vi "My Nonlinear Curve Fit TRDL bounds.vi"(0 "Y":dbl[](array[numeric]), 1 "f(x,a)":T5, 2 "data":variant, 5 "X":dbl[](array[numeric]), 7 "Weight":dbl[](array[numeric]), 9 "initial parameters":dbl[](array[numeric]), 11 "error in (no error)":errorcluster, 12 "Termination Criteria":T6={"Max Iterations"=0, "Max Function Calls"=0, "Max Time"=1000.0, "Function Tolerance"=1e-06, "Parameter Tolerance"=1e-06, "Gradient Tolerance"=0.0, "Min Lambda"=1e-06, "Max Lambda"=1e-06, "Initial Tick Count"=0}, 13 "parameter bounds":T4, 14 "method":T3 items=["Least Square", "Least Absolute Residual", "Bisquare"]) -> (3 "Fit Aborted?":bool, 4 "best nonlinear fit":dbl[](array[numeric]), 6 "best fit parameters":dbl[](array[numeric]), 8 "covariance":T7, 10 "Fit Statistics":T1={"# Iterations"=0, "# Function Calls"=0, "Chi2"=0.0, "Chi2/DOF"=0.0, "Fit Convergence Criterion"=enum."Continue", "Gradient"=0.0, "|Delta Chi 2|"=0.0, "|Delta Chi 2|/Chi 2"=0.0, "Max |Delta a| /|a|"=0.0, "Lambda"=-1.0}, 15 "error out":errorcluster)   [LabVIEW 2021, in "Fits.lvlib"]
uses:
  Fits.lvlib
  <vilib>/gmath/NumericalOptimization/LM_output select.ctl
  <vilib>/gmath/NI_Gmath.lvlib
  <vilib>/Analysis/NI_AALBase.lvlib
  <vilib>/gmath/NumericalOptimization/LM model function reference.ctl
  <vilib>/gmath/NumericalOptimization/LM model function.ctl
  Fit Statistics v3.ctl
  Abort Fit Global.vi
  <vilib>/Analysis/baseanly.llb/Real Inverse Matrix.vi
  Error/Error.lvlib
  Convergence Criteria.ctl
  <vilib>/Analysis/Matrix/Datatypes/RealMatrix.ctl
  <vilib>/Analysis/Matrix/NI_Matrix.lvlib
  <vilib>/Analysis/6fits.llb/Curve Fitting Criteria.ctl
  <vilib>/Analysis/NI_AALPro.lvlib
  My Fit Stopping Criteria.ctl
panel:
  out "Waveform Graph":dbl[](graph)
  in  "Delay (ms)":i32
  in  "Debug":bool
  out "Parameters Chart":dbl[][](graph)
  out "Function & Fit Graph":cluster{"New Coefficients":dbl[]}[](graph)
  in  "TR update constants":cluster{"h1":dbl, "h2":dbl, "a1":dbl, "a2":dbl}={"h1"=0.0001, "h2"=0.99, "a1"=0.25, "a2"=3.5}
  out "number of function calls":i32
  out "residue":dbl
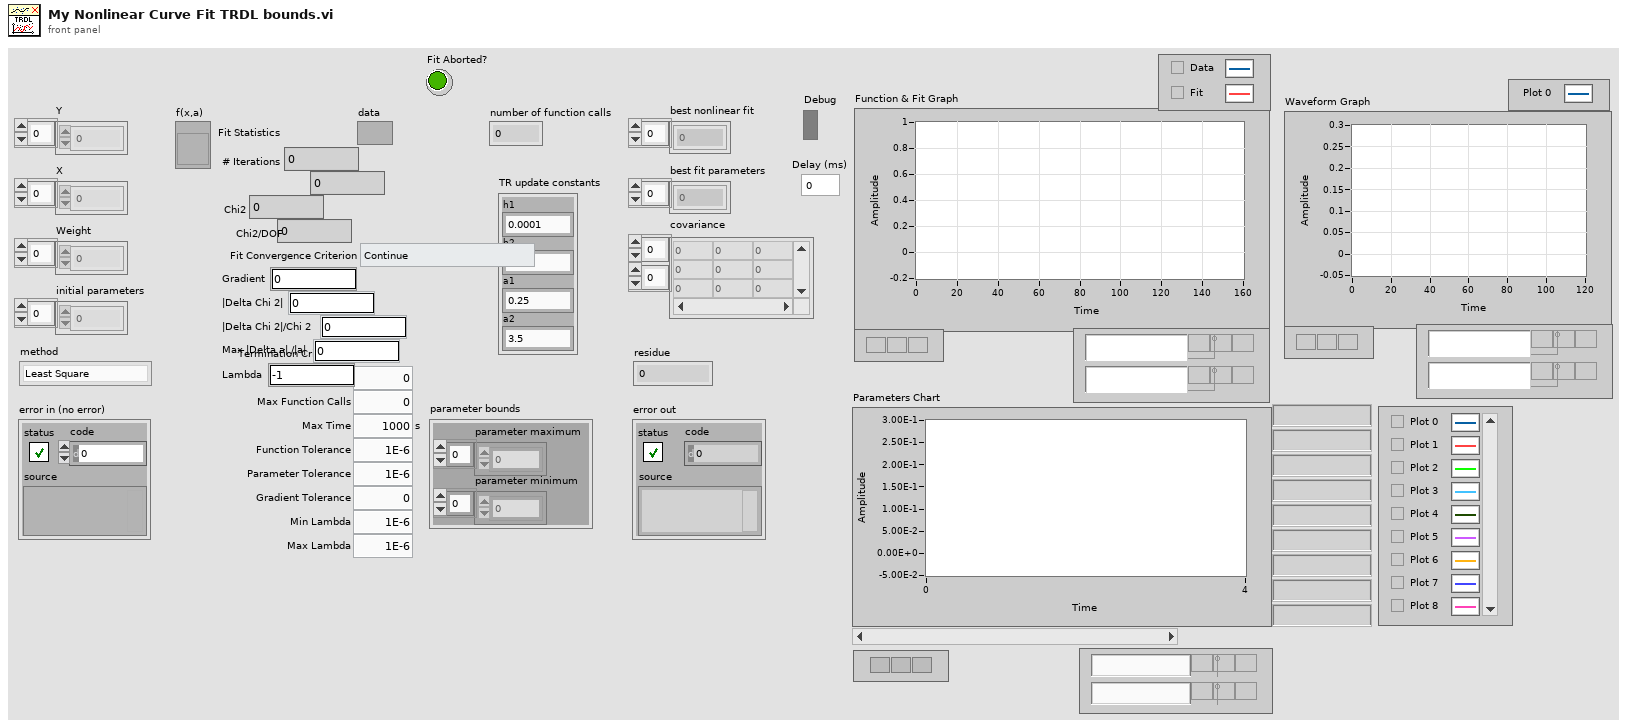
[diagram p1: front panel]
types:
  T1 = typedef "Fits.lvlib/Fit Statistics v2.ctl" = cluster{"# Iterations":i32, "# Function Calls":i32, "Chi2":dbl, "Chi2/DOF":dbl, "Fit Convergence Criterion":T2, "Gradient":dbl, "|Delta Chi 2|":dbl, "|Delta Chi 2|/Chi 2":dbl, "Max |Delta a| /|a|":dbl, "Lambda":dbl}
  T2 = typedef "Fits.lvlib/Convergence Criteria.ctl" = enum16{"Continue", "Tolerances Exceeded", "Max Time Exceeded", "Max Iterations Exceeded", "Max Function Evaluations Exceeded", "Scale Range Exceeded"}
  T3 = typedef "NI_AALPro.lvlib/Curve Fitting Criteria.ctl" = u16
  T4 = cluster{"parameter minimum":dbl[], "parameter maximum":dbl[]}
  T5 = typedef "NI_Gmath.lvlib/LM model function reference.ctl" = refnum<vi>
  T6 = typedef "Fits.lvlib/My Fit Stopping Criteria.ctl" = cluster{"Max Iterations":i32, "Max Function Calls":i32, "Max Time":dbl[unit], "Function Tolerance":dbl, "Parameter Tolerance":dbl, "Gradient Tolerance":dbl, "Min Lambda":dbl, "Max Lambda":dbl, "Initial Tick Count":u32}
  T7 = typedef "NI_Matrix.lvlib/RealMatrix.ctl" = dbl[][]
  T8 = typedef "NI_Gmath.lvlib/LM model function.ctl" = cluster{"f(x,a)":T5, "data":variant}
  T9 = typedef "NI_Gmath.lvlib/LM_output select.ctl" = cluster{"model function":bool, "gradient":bool}
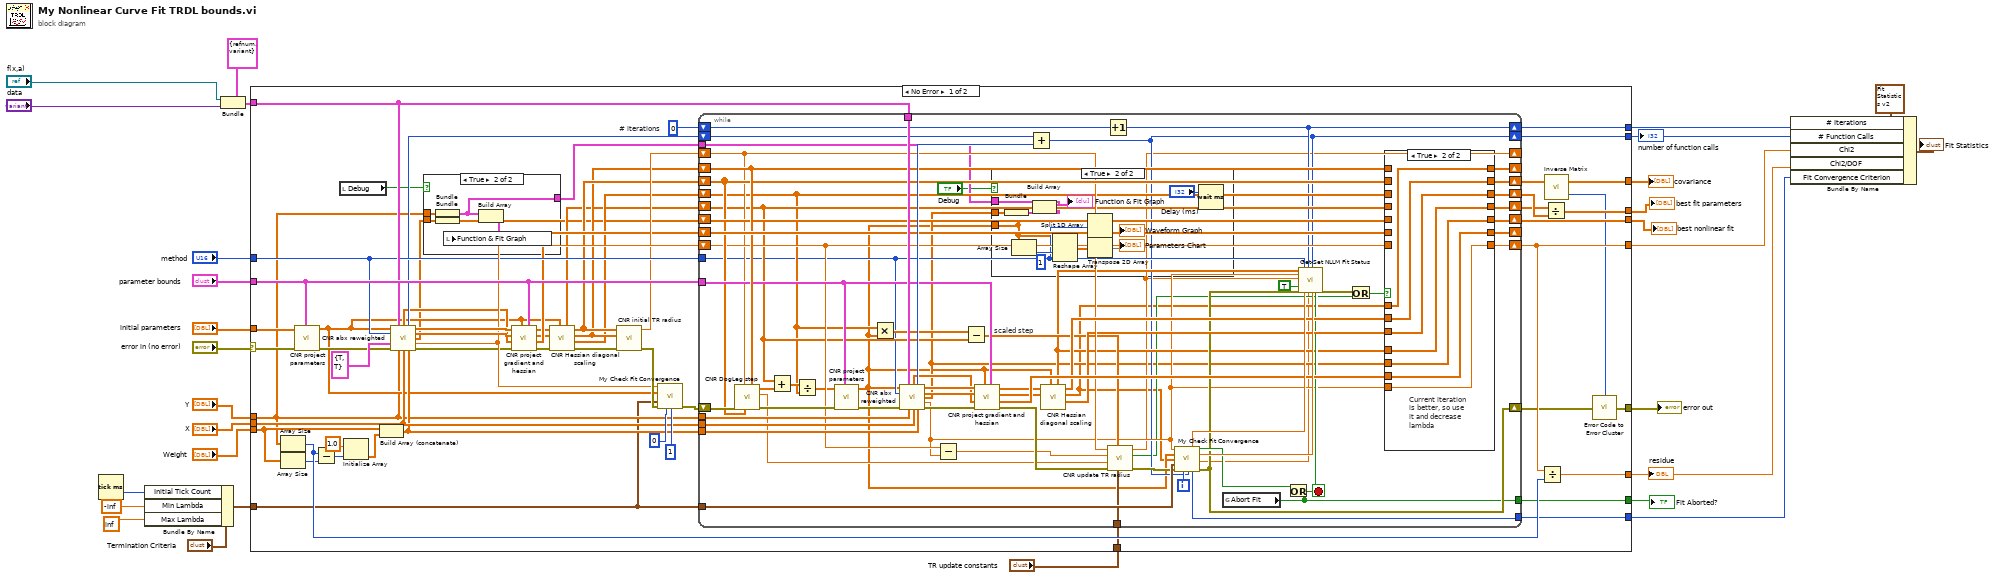
[diagram p0: block diagram]
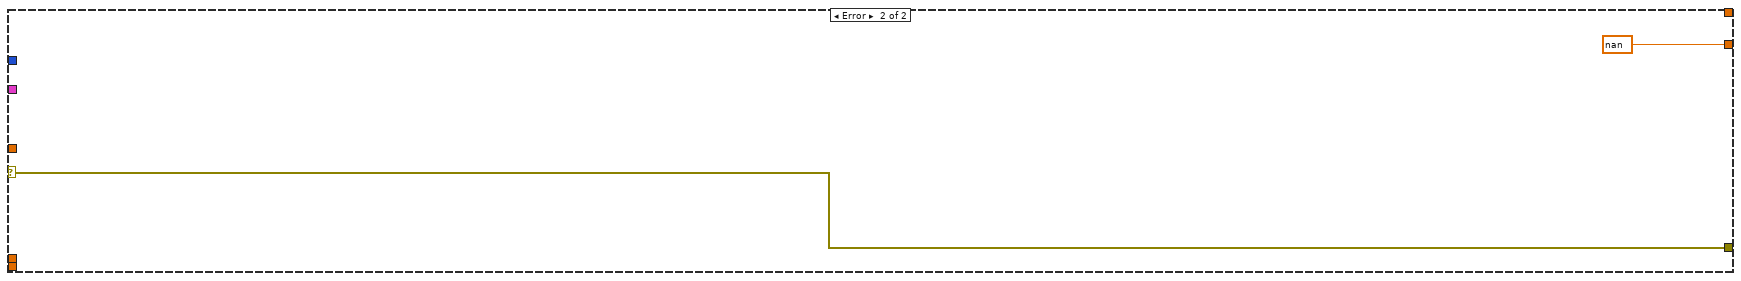
[diagram p5: hidden frame]
diagram:
  n1 = Tick Count (ms)() -> (millisecond timer value=w5:u32)
  n2 = Bundle By Name(cluster="Termination Criteria", "Initial Tick Count"=w5, "Min Lambda"=-inf ("min lambda"), "Max Lambda"=inf ("max lambda")) -> (w17:T6)
  n3 = Bundle(cluster=T8 {"f(x,a)"=refnum, "data"=variant} ("model function"), "f(x,a)"="f(x,a)", "data"="data") -> (w18:T8)
  n4 = case shown="No Error" "error in (no error)" {
    selector: "error in (no error)" -> [w71 w188]
    tunnel: [w43 _] -> w29
    tunnel: [w85 _] -> w8
    tunnel: "initial parameters" -> [w47 _]
    tunnel: [w57 _] -> w27
    tunnel: [w72 _] -> w26
    tunnel: "Weight" -> [w80 _]
    tunnel: "Y" -> [w36 _]
    tunnel: w17 -> [w34 _]
    tunnel: "X" -> [w59 _]
    tunnel: [w32 w188] -> w22
    tunnel: w18 -> [w65 _]
    tunnel: [w76 _] -> w9
    tunnel: "parameter bounds" -> [w70 _]
    tunnel: "method" -> [w64 _]
    tunnel: "TR update constants" -> [w56 _]
    tunnel: [w41 _] -> w11
    tunnel: [w40 nan ("chiSqr")] -> w7
    tunnel: [w39 _] -> w6
    tunnel: [w30 _] -> w1
    frame No Error {
      w42 = 0  # # iterations
      n5 = Array Size(array=w36) -> (size(s)=w86:i32)
      n6 = Array Size(array=w80) -> (size(s)=w83:i32)
      n7 = call <vilib>:"CNR project parameters.vi"("bounds"=w70, "error in"=w71, "parameters"=w47) -> ("error out"=w63:errorcluster, "projected parameters"=w46:dbl[])  [unwired: 7 out]
      n8 = Subtract(x=w86, y=w83) -> (x-y=w82:i32)
      n9 = local read "Debug"() -> (w38:bool)
      n10 = Initialize Array(1.0, w82) -> (w81:dbl[])
      n11 = Build Array (concatenate)(w80, w81) -> (w58:dbl[])
      n12 = call <vilib>:"CNR abx reweighted.vi"("parameters"=w46, "model function"=w65, "method"=w64, "output control"=T9 {"model function"=TRUE, "gradient"=TRUE}, "error in (no error)"=w63, "Y"=w36, "X"=w59, "Weight"=w58) -> ("Jacobian"=w54:T7, "number of function calls"=w62:i32, "Hessian"=w69:T7, "gradient"=w68:dbl[], "best fit"=w37:dbl[], "chiSqr"=w67:dbl, "error out"=w61:errorcluster)  [unwired: 1 in]
      n13 = case shown="True" w38 {
        tunnel: w37 -> [_ w90]
        tunnel: w36 -> [_ w89]
        tunnel: [_ w87] -> w35
        frame False {
        }
        frame True {
          n14 = Bundle("Y"=w89) -> (w87:cluster{"Y":dbl[]})  [unwired: 1 in]
          n15 = Bundle("best fit"=w90) -> (w91:cluster{"best fit":dbl[]})  [unwired: 1 in]
          n16 = Build Array(w87, w91) -> (w88:cluster{"best fit":dbl[]}[])
          n17 = local write "Function & Fit Graph"(w88) -> ()
        }
      }
      n18 = call <vilib>:"CNR project gradient and hessian.vi"("bounds"=w70, "projected parameters"=w46, "error in"=w61, "Jacobian"=w54, "gradient"=w68, "Hessian"=w69) -> ("error out"=w60:errorcluster, "projected jacobian"=w53:T7, "projected gradient"=w50:dbl[], "projected Hessian"=w52:T7)  [unwired: 1 in, 1 out]
      n19 = call <vilib>:"CNR Hessian diagonal scaling.vi"("parameters"=w46, "gradient"=w50, "Hessian"=w52) -> ("D"=w48:dbl[], "scaled gradient"=w49:dbl[], "scaled Hessian"=w51:T7, "scaled parameters"=w45:dbl[])  [unwired: 5 out]
      n20 = call <vilib>:"CNR initial TR radius.vi"("error in"=w60, "g"=w49, "H"=w51) -> ("error out"=w74:errorcluster, "initial TR radius"=w55:dbl)  [unwired: 7 out]
      n21 = call "My Check Fit Convergence.vi"("Chi 2"=w67, "Parameters"=w46, "my stopping criteria"=w34, "Error In"=w74, "current iteration"=0, "number of function evaluations"=1) -> ("error out"=w79:errorcluster)  [unwired: 2 in, 7 out]
      n22 = while {
        tunnel: w59 -> [w158]
        tunnel: w36 -> [w134]
        shift-left: w67 -> [w129]
        shift-right: [w151] -> w40
        shift-left: w45 -> [w120]
        shift-right: [w148] -> w44
        shift-left: w55 -> [w121]
        shift-right: [w100] -> _
        shift-right: [w110] -> w33
        shift-left: w79 -> [w149]
        tunnel: w65 -> [w157]
        tunnel: w34 -> [w153]
        shift-right: [w104] -> w76
        shift-left: w62 -> [w156]
        shift-right: [w155] -> w57
        shift-left: w37 -> [w133]
        shift-right: [w152] -> _
        shift-left: w53 -> [w147]
        tunnel: w58 -> [w142]
        shift-right: [w146] -> w75
        shift-left: w48 -> [w114]
        tunnel: w70 -> [w135]
        shift-right: [w145] -> _
        shift-left: w49 -> [w143]
        shift-right: [w144] -> w73
        shift-left: w51 -> [w131]
        tunnel: w64 -> [w106]
        tunnel: w56 -> [w132]
        shift-right: [w105] -> w41
        shift-left: w42 -> [w112]
        tunnel: [w99] -> w39
        tunnel: w35 -> [w97]
        tunnel: [w92] -> w30
        i -> [w154]
        stop <- w109 stop-if-true
        # "scaled step"
        n23 = call <vilib>:"CNR DogLeg step.vi"("gradient"=w143, "Hessian"=w131, "TR radius"=w121, "error in (no error)"=w149) -> ("error out"=w141:errorcluster, "L(0)-L(hdl)\npredicted change"=w124:dbl, "x step"=w118:dbl[])  [unwired: 3 in, 2 out]
        n24 = Add(x=w120, y=w118) -> (x+y=w117:dbl[])
        n25 = Divide(x=w117, y=w114) -> (x/y=w116:dbl[])
        n26 = call <vilib>:"CNR project parameters.vi"("bounds"=w135, "error in"=w141, "parameters"=w116) -> ("error out"=w140:errorcluster, "projected parameters"=w95:dbl[])  [unwired: 7 out]
        n27 = Multiply(x=w114, y=w95) -> (x*y=w113:dbl[])
        n28 = call <vilib>:"CNR abx reweighted.vi"("parameters"=w95, "model function"=w157, "method"=w106, "error in (no error)"=w140, "Y"=w134, "X"=w158, "Weight"=w142) -> ("Jacobian"=w123:T7, "number of function calls"=w159:i32, "Hessian"=w137:T7, "gradient"=w136:dbl[], "best fit"=w98:dbl[], "chiSqr"=w107:dbl, "error out"=w139:errorcluster)  [unwired: 2 in]
        n29 = Subtract(x=w129, y=w107) -> (x-y=w125:dbl)
        n30 = Subtract(x=w113, y=w120) -> (x-y=w115:dbl[])
        n31 = call <vilib>:"CNR project gradient and hessian.vi"("bounds"=w135, "projected parameters"=w95, "error in"=w139, "Jacobian"=w123, "gradient"=w136, "Hessian"=w137) -> ("error out"=w138:errorcluster, "projected jacobian"=w130:T7, "projected gradient"=w126:dbl[], "projected Hessian"=w128:T7)  [unwired: 1 in, 1 out]
        n32 = case shown="True" "Debug" {
          tunnel: w98 -> [_ w169]
          tunnel: w97 -> [_ w168]
          tunnel: w95 -> [_ w163]
          frame False {
          }
          frame True {
            w164 = 1 ("dimension size")
            n33 = Bundle("best fit"=w169) -> (w172:cluster{"best fit":dbl[]})  [unwired: 1 in]
            n34 = Array Size(array=w163) -> (size(s)=w171:i32)
            n35 = Build Array(w168, w172) -> (→"Function & Fit Graph":cluster{"best fit":dbl[]}[])
            n36 = Reshape Array(w163, w171, w164) -> (w170:dbl[][])
            n37 = Split 1D Array(array=w163, index=w164) -> (second subarray=→"Waveform Graph":dbl[])  [unwired: 1 out]
            n38 = Transpose 2D Array(2D array=w170) -> (transposed array=→"Parameters Chart":dbl[][])
            n39 = Wait (ms)(milliseconds to wait="Delay (ms)") -> ()  [unwired: 1 out]
          }
        }
        n40 = Add(x=w156, y=w159) -> (x+y=w104:i32)
        n41 = call <vilib>:"CNR Hessian diagonal scaling.vi"("parameters"=w95, "gradient"=w126, "Hessian"=w128) -> ("D"=w119:dbl[], "scaled gradient"=w94:dbl[], "scaled Hessian"=w127:T7, "scaled parameters"=w108:dbl[])  [unwired: 5 out]
        n42 = Increment(x=w112) -> (x+1=w105:i32)
        n43 = call <vilib>:"CNR update TR radius.vi"("TR update constants"=w132, "step"=w115, "error in (no error)"=w138, "L(0)-L(p_dl)"=w124, "F(x)-F(x+p)"=w125, "TR Radius"=w121) -> ("error out"=w150:errorcluster, "step OK?"=w102:bool, "TR Radius out"=w100:dbl)  [unwired: 3 out]
        n44 = call "My Check Fit Convergence.vi"("Chi 2"=w107, "Parameters"=w95, "gradient"=w94, "my stopping criteria"=w153, "Error In"=w150, "current iteration"=w154, "number of function evaluations"=w104) -> ("|Delta Chi 2|/Chi 2"=w161:dbl, "stop?"=w122:bool, "|Delta Chi 2|"=w160:dbl, "Max |Delta a| /|a|"=w93:dbl, "Convergence Criterium Reached"=w92:T2, "error out"=w110:errorcluster)  [unwired: 1 in, 2 out]
        n45 = global read "Abort Fit Global.vi" "Abort Fit"() -> (w99:bool)
        n46 = Or(x=w122, y=w99) -> (x .or. y?=w109:bool)
        n47 = call "Get-Set NLLM Fit Status.vi"("Fit Parameters"=w108, "chiSqr"=w107, "Lambda"=w100, "Get(F)/Set"=TRUE, "Error In"=w110, "NL Fit Method"=w106, "|Delta Chi 2|/Chi 2"=w161, "# Iterations"=w105, "Max |Delta a| /|a|"=w93, "# Function Calls"=w104, "|Delta Chi 2|"=w160, "Done"=w109) -> ("Error Out"=w103:errorcluster)  [unwired: 6 in, 1 out]
        n48 = Or(x=w103, y=w102) -> (x .or. y?=w101:bool)
        n49 = case shown="True" w101 {
          tunnel: w108 -> [_ w180]
          tunnel: w120 -> [w179 _]
          tunnel: [w179 w180] -> w148
          tunnel: w129 -> [w178 _]
          tunnel: w107 -> [_ w186]
          tunnel: [w178 w186] -> w151
          tunnel: w133 -> [w177 _]
          tunnel: [w177 w184] -> w155
          tunnel: w147 -> [w176 _]
          tunnel: [w176 w185] -> w152
          tunnel: w130 -> [_ w185]
          tunnel: w98 -> [_ w184]
          tunnel: w114 -> [w175 _]
          tunnel: [w175 w181] -> w146
          tunnel: w143 -> [w174 _]
          tunnel: w131 -> [w173 _]
          tunnel: [w174 w183] -> w145
          tunnel: [w173 w182] -> w144
          tunnel: w94 -> [_ w183]
          tunnel: w127 -> [_ w182]
          tunnel: w119 -> [_ w181]
          frame False {
            # "Previous iteration\nis better, so keep\nit and increase \nlambda"
          }
          frame True {
            # "Current iteration\nis better, so use\nit and decrease \nlambda"
          }
        }
      }
      n50 = Divide(x=w40, y=w86) -> (x/y=w85:dbl)
      n51 = Divide(x=w44, y=w75) -> (x/y=w43:dbl[])
      n52 = call-poly <vilib>:"Inverse Matrix.vi"("Input Matrix"=w73) -> ("error"=w31:i32, "Inverse Matrix"=w72:T7)  [unwired: 1 in]
      n53 = call "Error Code to Error Cluster.vi"("Error Code"=w31, "Error In"=w33) -> ("Error Out"=w32:errorcluster)  [unwired: 13 in]
    }
    frame Error {
    }
  }
  "residue" <- w8
  "best fit parameters" <- w29
  "best nonlinear fit" <- w27
  "error out" <- w22
  "covariance" <- w26
  "number of function calls" <- w9
  "Fit Aborted?" <- w6
  n54 = Bundle By Name(cluster=T1 {"# Iterations"=0, "# Function Calls"=0, "Chi2"=0.0, "Chi2/DOF"=0.0, "Fit Convergence Criterion"=enum."Continue", "Gradient"=0.0, "|Delta Chi 2|"=0.0, "|Delta Chi 2|/Chi 2"=0.0, "Max |Delta a| /|a|"=0.0, "Lambda"=-1.0} ("Fit Statistics"), "# Iterations"=w11, "# Function Calls"=w9, "Chi2"=w7, "Chi2/DOF"=w8, "Fit Convergence Criterion"=w1) -> (→"Fit Statistics":T1)
